vi "Write_BIn.vi"(0 "Refnum in":refnum<k21>, 1 "Estados":bool[](array[boolean]), 5 "error in (no error)":errorcluster) -> (14 "Refnum out":refnum<k21>, 19 "error out":errorcluster)   [LabVIEW 2013]
uses:
  <vilib>/DAQmx/write.llb/DAQmx Write (Digital U32 1Chan 1Samp).vi
  <vilib>/DAQmx/miscellaneous.llb/DAQmx Fill In Error Info.vi
panel:
  out "number":u32
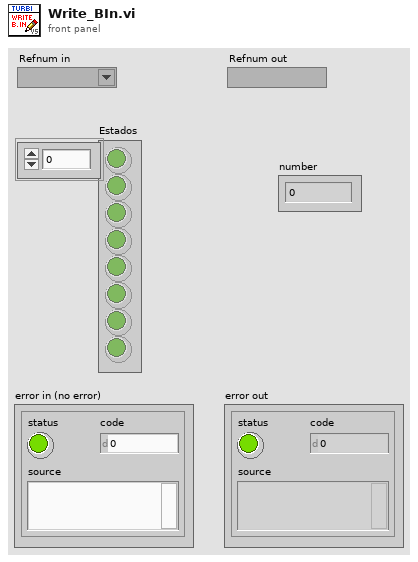
[diagram p1: front panel]
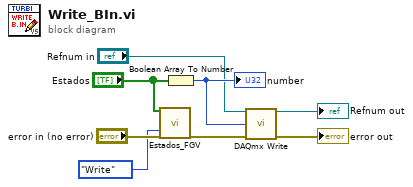
[diagram p0: block diagram]
diagram:
  n1 = call "Estados_FGV.vi"("Estados_IN"="Estados", "Opción"=enum16{"Write", "Read"}."Write", "Error In"="error in (no error)") -> ("Error Out"=w3:errorcluster)  [unwired: 15 in, 1 out]
  n2 = Boolean Array To Number(Boolean array="Estados") -> (number=w6:u32)
  "number" <- w6
  n3 = call-poly <vilib>:"DAQmx Write.vi"("task/channels in"="Refnum in", "data"=w6, "error in"=w3) -> ("task out"=→"Refnum out":refnum<k21>, "error out"=→"error out":errorcluster)  [unwired: 10 in, 1 out]
